vi "Remove Local Chassis.vi"(8 "error in":errorcluster, 11 "local chassis ref":T1 format="%.0x") -> (0 "error out":errorcluster)   [LabVIEW 2020, in "Scan Engine Scripting.lvlib"]
doc: "Removes the specified local chassis from the Scan Engine and EtherCAT custom device."
uses:
  Scan Engine Scripting.lvlib
  <vilib>/NI VeriStand/Custom Device API/Custom Device Item Ref.ctl
  Scan Engine Dependencies.llb/Scan Engine GUIDs.vi
  Scan Engine Dependencies.llb/Scan Engine Custom Device.lvlib
  <vilib>/NI VeriStand/Custom Device API/Custom Device API.lvlib
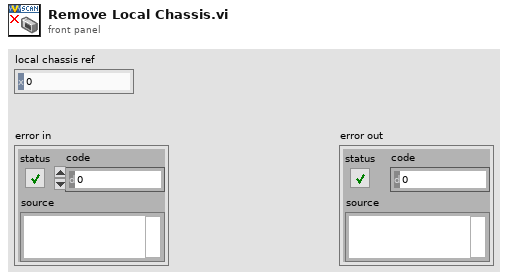
[diagram p1: front panel]
types:
  T1 = typedef "Custom Device API.lvlib/Custom Device Item Ref.ctl" = u64
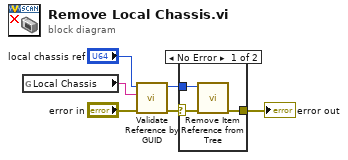
[diagram p0: block diagram]
diagram:
  n1 = global read "Scan Engine GUIDs.vi" "Local Chassis"() -> (w4:string)
  n2 = call "Validate Reference by GUID.vi"("error in"="error in", "GUID"=w4, "item in"="local chassis ref") -> ("error out"=w6:errorcluster, "item out"=w5:T1)  [unwired: 7 in]
  n3 = case shown="No Error" w6 {
    selector: w6 -> [w8 w10]
    tunnel: w5 -> [w9 _]
    tunnel: [w7 w10] -> w1
    frame No Error {
      n4 = call "Remove Item Reference from Tree.vi"("error in"=w8, "item ref"=w9) -> ("error out"=w7:errorcluster)  [unwired: 8 in, 1 out]
    }
    frame Error {
    }
  }
  "error out" <- w1
